vi "Add Custom Device_Pre and Post Init VI.vi"(8 "error in (no error)":errorcluster, 10 "Custom Device Settings":T2, 11 "System Definition Ref":T1) -> (0 "error out":errorcluster, 3 ".NET Refnum out":T1)   [LabVIEW 2019, in "Simple SysDef API.lvlib"]
uses:
  <userlib>/SimpleSysDef/Simple SysDef API.lvlib
  <userlib>/SimpleSysDef/_SubVIs/System Definition Reference.ctl
  NationalInstruments.VeriStand.SystemDefinitionAPI
  <userlib>/SimpleSysDef/_SubVIs/Add Custom Device_Settings.ctl
  <userlib>/SimpleSysDef/_SubVIs/Add Custom Device.vi
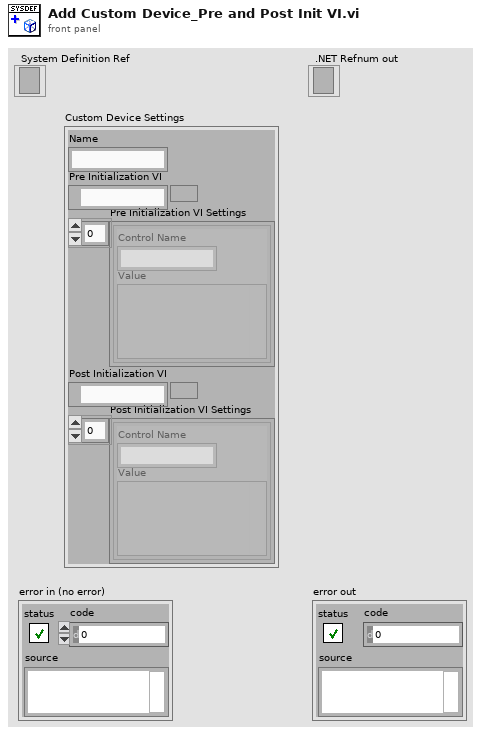
[diagram p1: front panel]
types:
  T1 = typedef "Simple SysDef API.lvlib/System Definition Reference.ctl" = refnum<k24>
  T2 = cluster{"Name":string, "Pre Initialization VI":path, "Pre Initialization VI Settings":cluster{"Control Name":string, "Value":variant}[], "Post Initialization VI":path, "Post Initialization VI Settings":cluster{"Control Name":string, "Value":variant}[]}
  T3 = typedef "Simple SysDef API.lvlib/Add Custom Device_Settings.ctl" = cluster{"Name":string, "customDevice":refnum<k24>}
  T4 = cluster{"Control Name":string, "Value":variant}[]
  T5 = typedef "Simple SysDef API.lvlib/Custom Device Control Name and Ref.ctl" = cluster{"customDevice":refnum<k24>, "Control Name":string}
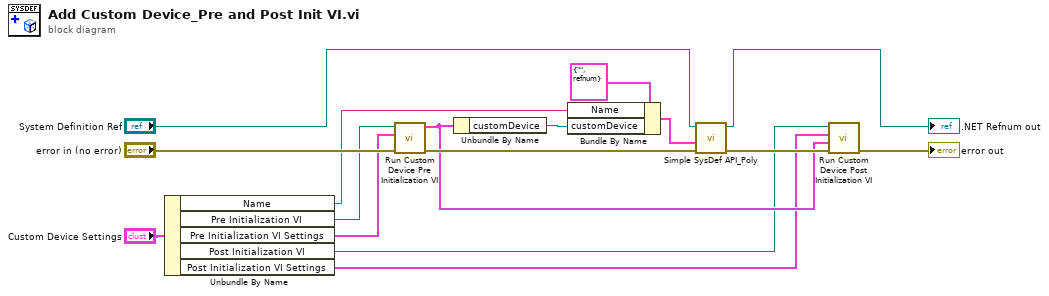
[diagram p0: block diagram]
diagram:
  n1 = Unbundle By Name("Custom Device Settings") -> ("Name"=w5:string, "Pre Initialization VI"=w4:path, "Pre Initialization VI Settings"=w3:T4, "Post Initialization VI"=w2:path, "Post Initialization VI Settings"=w1:T4)
  n2 = call <userlib>:"Run Custom Device Pre Initialization VI.vi"("error in (no error)"="error in (no error)", "Settings"=w3, "Pre Initialization VI"=w4) -> ("error out"=w11:errorcluster, "Custom Device Ref"=w6:T5)  [unwired: 7 in]
  n3 = Unbundle By Name(w6) -> ("customDevice"=w7:refnum<k24>)
  n4 = Bundle By Name(cluster=T3 {"Name"="", "customDevice"=refnum} ("Settings"), "Name"=w5, "customDevice"=w7) -> (w9:T3)
  n5 = call-poly <userlib>:"Simple SysDef API_Poly.vi"("error in (no error)"=w11, "Settings"=w9, "SysDef Ref"="System Definition Ref") -> ("error out"=w8:errorcluster, "SysDef Ref Out"=→".NET Refnum out":T1)  [unwired: 6 in, 1 out]
  n6 = call <userlib>:"Run Custom Device Post Initialization VI.vi"("error in (no error)"=w8, "Custom Device Ref"=w6, "Settings"=w1, "Post Initialization VI"=w2) -> ("error out"=→"error out":errorcluster)  [unwired: 7 in]
